vi "Main.vi"() -> ()   [LabVIEW 2010]
uses:
  <vilib>/Platform/storage/lvStorage.llb/xStorage/Open Data Storage/Open Data Storage.xnode
  <vilib>/Platform/storage/lvStorage.llb/xStorage/Set Properties/Set Properties.xnode
  <vilib>/Platform/storage/lvStorage.llb/xStorage/Write Data/Write Data.xnode
  <vilib>/Platform/storage/Storage.llb/usiOverwriteOptions.ctl
  <vilib>/Platform/storage/Storage.llb/usiSequenceRepresentation.ctl
  <vilib>/Platform/storage/lvStorage.llb/xStorage/Close Data Storage/Close Data Storage.xnode
  <instrlib>/Tektronix DPO MSO 2000 4000 Series/Public/Data/Read (Single Waveform).vi
  <instrlib>/Tektronix DPO MSO 2000 4000 Series/Public/Data/Read (Multiple Waveforms).vi
  <instrlib>/Tektronix DPO MSO 2000 4000 Series/Public/Configure/Configure Math (Dual).vi
  <vilib>/Platform/storage/lvStorage.llb/_openStorageWithRootAutoDetect.vi
  <vilib>/Platform/storage/lvStorage.llb/xStorage/xStorageSupp/ErrorOut.vi
  <vilib>/Platform/storage/Storage.llb/__savePropString.vi
  <vilib>/Platform/storage/Storage.llb/__savePropTime.vi
  <vilib>/Platform/storage/lvStorage.llb/_createOrGetByNameExplicitChildObject.vi
  <vilib>/Platform/storage/lvStorage.llb/_prepDDT.vi
  <vilib>/Platform/storage/lvStorage.llb/_getChannelNameFromDDT.vi
  <vilib>/Platform/storage/lvStorage.llb/_saveDDT.vi
  <vilib>/Platform/storage/Storage.llb/Get Object Info.vi
  <vilib>/Platform/storage/Storage.llb/__closeStorageFromObject.vi
  <instrlib>/Tektronix DPO MSO 2000 4000 Series/Tektronix DPO MSO 2000 4000 Series.lvlib
  user32.dll
  shell32.dll
panel:
  out "error out 8":errorcluster
  in  "stop 2":bool
  out "error out 7":errorcluster
  out "error out 6":errorcluster
  in  "stop":bool
  out "Array 5":dbl[](array[numeric])
  out "Array 4":dbl[](array[numeric])
  out "Array 3":dbl[](array[numeric])
  out "Array 2":dbl[](array[numeric])
  out "error out 5":errorcluster
  out "error out 4":errorcluster
  out "ERROR":bool
  in  "Parameters":string
  out "Array":string[](array[string])
  out "error out 2":errorcluster
  out "error out":errorcluster
  out "down":bool
  out "up":bool
  out "DOWN":dbl
  out "UP":dbl
  in  "Error Range":dbl min=0.0 max=5.0 step=0.1 format="%#.3g%"
  in  "Port to test":u16(ring) items=["AMB 1", "AMB 2", "AMB 3", "AMB 4", "AMB 5", "AMB 18"]
  in  "Assembled by":string="Alexis Ibarra"
  in  "ABM-S/N":string
  in  "IP Addres":string
  in  "Tab Control":T1(tab)
  in  "Start TE TEST":bool
  out "TIMA":waveform(dbl)(graph)
  out "TIMB":waveform(dbl)(graph)
  out "Differential Signal":waveform(dbl)(graph)
  out "TE Signals":waveform(dbl)[](graph)
  in  "Maximum Time (10000ms)":u32=20000
  in  "Channel B (1: Channel 2)":u16(ring)=1 items=["Channel 1", "Channel 2", "Channel 3", "Channel 4", "Math", "Reference 1", "Reference 2", "Reference 3", "Reference 4"]
  in  "Channel A (0: Channel 1)":u16(ring) items=["Channel 1", "Channel 2", "Channel 3", "Channel 4", "Math", "Reference 1", "Reference 2", "Reference 3", "Reference 4"]
  out "TE Periode":dbl
  out "TE Average":dbl
  out "TE STATUS":string
  out "TE Amplitude":dbl format="%#_gv"
  in  "Start CCT TEST":bool
  out "TIMB 2":waveform(dbl)(graph)
  out "CAN Diferential":waveform(dbl)(graph)
  out "CAN+TIMB":waveform(dbl)[](graph)
  in  "Maximum Time (10000ms) t2":u32=20000
  in  "Channel B (1: Channel 2) 2":u16(ring)=1 items=["Channel 1", "Channel 2", "Channel 3", "Channel 4", "Math", "Reference 1", "Reference 2", "Reference 3", "Reference 4"]
  in  "Channel A (0: Channel 1) 2":u16(ring) items=["Channel 1", "Channel 2", "Channel 3", "Channel 4", "Math", "Reference 1", "Reference 2", "Reference 3", "Reference 4"]
  out "CCT Delay":dbl format="%^#_6gs"
  out "CCT Average":dbl format="%#_gms"
  out "CCT STATUS":string
  out "Amplitude":dbl format="%#_gv"
  in  "Start CSMT TEST":bool
  out "CAN+TIMB 2":waveform(dbl)(graph)
  out "TIMB 3":waveform(dbl)(graph)
  out "CAN Diferential 2":waveform(dbl)(graph)
  out "CSMT Averege":dbl
  out "CSMT Periode":dbl
  out "CSMT Status":string
  in  "Maximum Time (10000ms) 2":u32=20000
  in  "Channel B (1: Channel 2) 3":u16(ring)=1 items=["Channel 1", "Channel 2", "Channel 3", "Channel 4", "Math", "Reference 1", "Reference 2", "Reference 3", "Reference 4"]
  in  "Channel A (0: Channel 1) 3":u16(ring) items=["Channel 1", "Channel 2", "Channel 3", "Channel 4", "Math", "Reference 1", "Reference 2", "Reference 3", "Reference 4"]
  out "Amplitude":dbl format="%#_gv"
  in  "Start RESET TEST":bool
  out "RESA+RESB":waveform(dbl)[](graph)
  out "RESB":waveform(dbl)(graph)
  out "RESA":waveform(dbl)(graph)
  in  "Channel B (1: Channel 2) 4":u16(ring)=1 items=["Channel 1", "Channel 2", "Channel 3", "Channel 4", "Math", "Reference 1", "Reference 2", "Reference 3", "Reference 4"]
  in  "Channel A (0: Channel 1) 4":u16(ring) items=["Channel 1", "Channel 2", "Channel 3", "Channel 4", "Math", "Reference 1", "Reference 2", "Reference 3", "Reference 4"]
  in  "Maximum Time (10000ms) 3":u32=20000
  out "average":dbl
  out "STATUS":string
  out "Delay":dbl format="%^#_6g"
  out "Amplitude":dbl format="%#_gv"
  in  "AMBSI 1 SERIAL NUMBER":string
  out "Output":string
  in  "Start CM test":bool
  out "Error":string
  in  "?":bool
  in  "?":bool
  in  "Enter ABM Serial Number":string
  in  "Reports":i32(listbox)=-1
  out "output param":i32
  in  "error in":errorcluster
  out "error out 3":errorcluster
  in  "?":bool
  # "ABM Verification System"
  # "Copyrigth Alexis Ibarrra -  ALMA  Computing"
  # "TE Test"
  # "Can Control Timming"
  # "Can Signals Monitoring Timming"
  # "Reset Signal"
  # "Search Reports"
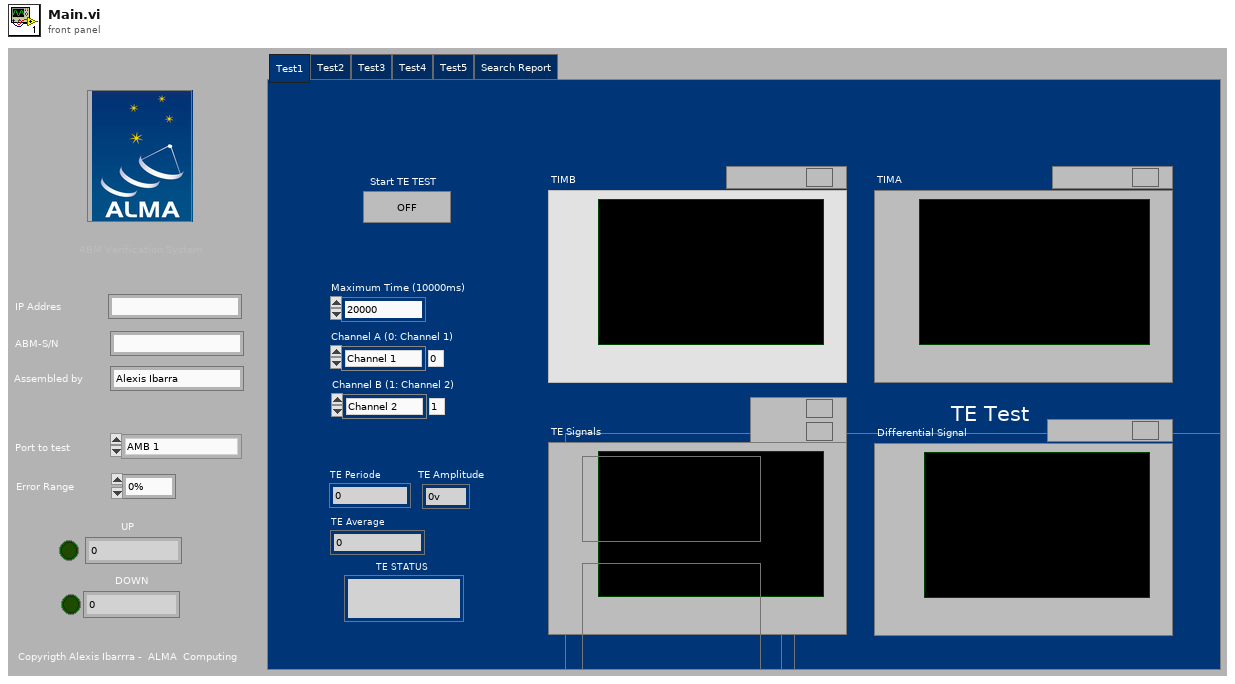
[diagram p1: front panel]
types:
  T1 = enum32{"Test1", "Test2", "Test3", "Test4", "Test5", "Search Report"}
  T2 = enum32{"invalid app kind", "Development System", "Run Time System", "Student Edition", "Embedded LabVIEW", "Evaluation", "Custom"}
  T3 = enum16{"open", "open or create", "create or replace", "create", "open (read only)"}
  T4 = enum16{"UPDATE", "READ", "QUERY", "CREATE CHILD", "CREATE", "CONNECT", "DISCONNECT"}
  T5 = typedef "usiOverwriteOptions.ctl" = enum16{"Append values", "Replace values at index", "Replace all values", "Append if timeline aligns"}
  T6 = typedef "usiSequenceRepresentation.ctl" = enum16{"explicit", "implicit"}
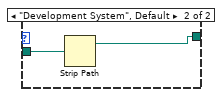
[diagram p3: hidden frame]
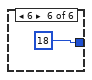
[diagram p8: hidden frame]
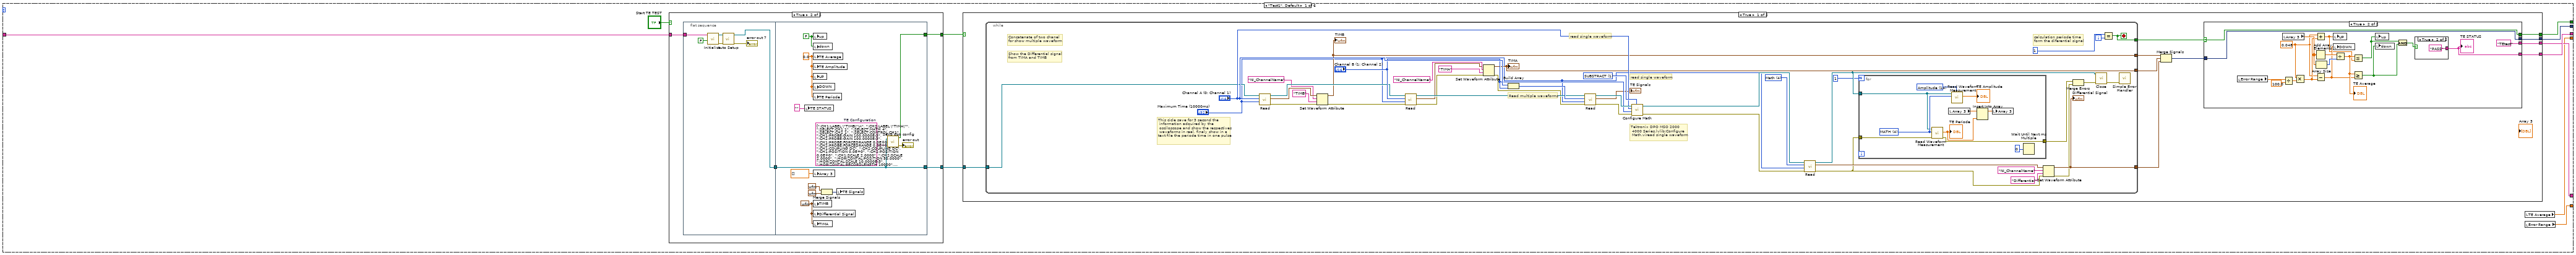
[diagram p9: hidden frame]
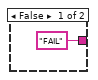
[diagram p11: hidden frame]
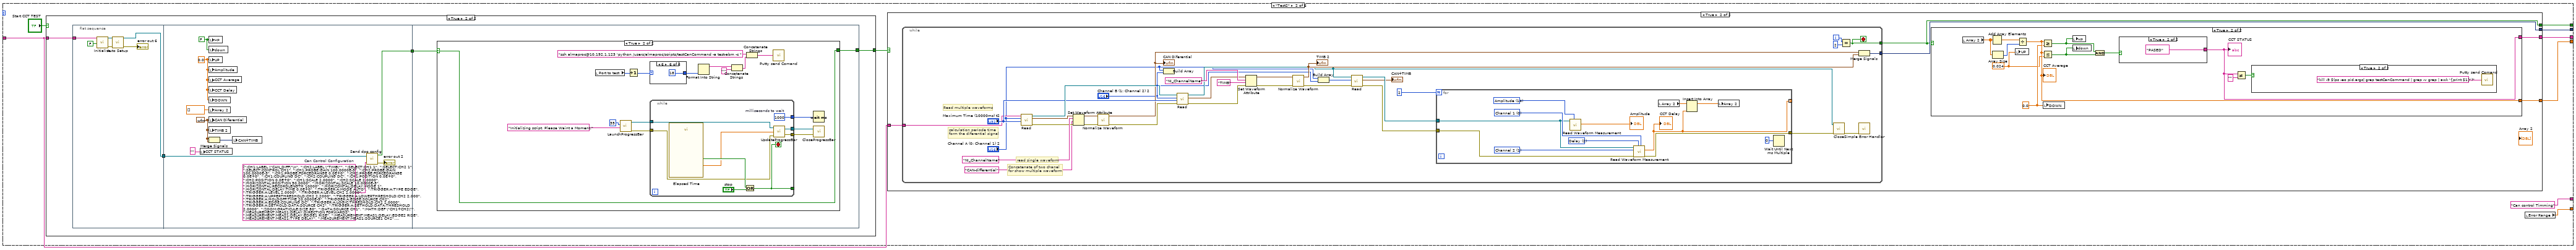
[diagram p14: hidden frame]
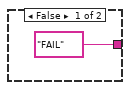
[diagram p18: hidden frame]
diagram:
  # "10.195.18.178"
  n1 = Concatenate Strings("TCPIP0::", "IP Addres", "::inst0::INSTR") -> (w2:string)
  n2 = case shown="\"Test3\"" "Tab Control" {
    tunnel: w2 -> [w19 w125 w251 w387 _ _]
    tunnel: [w18 w131 w254 w378 _ _] -> w1
    tunnel: [w17 w130 w257 w385 _ _] -> w7
    tunnel: [w16 w129 w255 w384 _ _] -> w6
    tunnel: [w12 w126 w252 w382 _ _] -> w5
    tunnel: [w13 w127 w253 w383 _ _] -> w4
    tunnel: [w15 "Can control Timming" "Can SIgnal Monitoring Timming" "Reset  test" _ _] -> w3
    frame "Test1", Default {
      n3 = case shown="True" "Start TE TEST" {
        tunnel: w19 -> [_ w105]
        tunnel: [_ w102] -> w20
        tunnel: [_ w103] -> w14
        frame False {
        }
        frame True {
          n4 = flat-sequence {
            tunnel: w105 -> [w108]
            tunnel: [w107] -> w104
            tunnel: w104 -> [w115]
            tunnel: [w115] -> w103
            tunnel: [w112] -> w102
            frame #0 {
              n5 = call <instrlib>:"Initialize.vi"("Reset (True)"=FALSE, "VISA resource name"=w108) -> ("error out"=w110:errorcluster, "VISA resource name out"=w109:refnum<visa-resource-name>)  [unwired: 8 in]
              n6 = call <instrlib>:"Auto Setup.vi"("error in (no error)"=w110, "VISA resource name"=w109) -> ("error out"=→"error out 7":errorcluster, "VISA resource name out"=w107:refnum<visa-resource-name>)  [unwired: 8 in]
            }
            frame #1 {
              w119 = waveform(dbl) {"t0"=timestamp(0 s since 1904-01-01), "dt"=1.0, "Y"=[]} ("Waveform")
              w123 = 0.0
              w117 = FALSE
              w114 = string[] [":CH1:LABEL \"TIMB\"\n", ":CH2:LABEL \"TIMA\"", ":SELECT:CH1 1", ":SELECT:MATH 4", ":SELECT:CH2 1", ":SELECT:CONTROL CH1", ":CH1:PROBE:GAIN 100.0000E-3", ":CH2:PROBE:GAIN 100.0000E-3", ":CH1:PROBE:FORCEDRANGE 0.0E+0", ":CH2:PROBE:FORCEDRANGE 0.0E+0", ":CH1:COUPLING DC", ":CH2:COUPLING DC", ":CH1:POSITION 0.0E+0", ":CH2:POSITION 0.0E+0", ":CH1:SCALE 2.0000", ":CH2:SCALE 2.0000", ":HORIZONTAL:POSITION 50.0000", ":HORIZONTAL:SCALE 10.0000E-3", ":HORIZONTAL:RECORDLENGTH 10000", ":HORIZONTAL:DELAY:MODE 1", ":HORIZONTAL:DELAY:TIME 0.0E+0", ":TRIGGER:A:MODE AUTO", ":TRIGGER:A:TYPE EDGE", ":TRIGGER:A:LEVEL 2.0000", ":TRIGGER:A:LEVEL:CH2 2.0000", ":TRIGGER:A:UPPERTHRESHOLD:CH2 2.2000", ":TRIGGER:A:LOWERTHRESHOLD:CH2 2.000", ":TRIGGER:A:HOLDOFF:TIME 20.0000E-9", ":TRIGGER:A:EDGE:SOURCE CH2", ":TRIGGER:A:EDGE:COUPLING DC", ":TRIGGER:A:LOGIC:THRESHOLD:CH2 2.0000", ":TRIGGER:A:SETHOLD:DATA:SOURCE CH2", ":TRIGGER:A:SETHOLD:DATA:THRESHOLD 2.0000", ":ZOOM:GRATICULE:SIZE 80", ":DATA:SOURCE CH2", ":MATH:POSITION -3.00E-3", ":MATH:SCALE 2.0000"]  # TE Configuration
              n7 = local write "TE STATUS"("" ("TE STATUS")) -> ()
              n8 = local write "up"(w117) -> ()
              n9 = local write "down"(w117) -> ()
              n10 = local write "TE Average"(w123) -> ()
              n11 = local write "TE Amplitude"(w123) -> ()
              n12 = local write "UP"(w123) -> ()
              n13 = local write "DOWN"(w123) -> ()
              n14 = local write "TE Periode"(w123) -> ()
              n15 = local write "Array 3"(dbl[] []) -> ()
              n16 = local write "TIMB"(w119) -> ()
              n17 = local write "Differential Signal"(w119) -> ()
              n18 = local write "TIMA"(w119) -> ()
              n19 = Merge Signals(waveform(dbl) {"t0"=timestamp(0 s since 1904-01-01), "dt"=1.0, "Y"=[]} ("Waveform"), waveform(dbl) {"t0"=timestamp(0 s since 1904-01-01), "dt"=1.0, "Y"=[]} ("Waveform")) -> (w122:dynamicdata)
              n20 = local write "TE Signals"(w122) -> ()
              n21 = call "Send dpo config.vi"("Array Configuration"=w114, "TCP/IP Addres"=w115) -> ("error out"=→"error out":errorcluster, "Exit"=w112:bool)  [unwired: 1 out]
            }
          }
        }
      }
      n22 = case shown="True" w20 {
        tunnel: w14 -> [w28 _]
        tunnel: [w24 _] -> w18
        tunnel: [w26 _] -> w17
        tunnel: [w23 _] -> w16
        tunnel: [w22 _] -> w15
        frame True {
          n23 = while {
            tunnel: [w65] -> w31
            tunnel: w28 -> [w80]
            tunnel: [w77] -> w29
            tunnel: [w69] -> w30
            tunnel: [w52] -> w25
            i -> [w55]
            stop <- w52 stop-if-true
            w61 = u16 4 items=["Channel 1", "Channel 2", "Channel 3", "Channel 4", "Math", "Reference 1", "Reference 2", "Reference 3", "Reference 4"] ("Channel (0: Channel 1)")
            w88 = u16 1 items=["ADD", "SUBSTRACT", "MULTIPLY", "DIVIDE"] ("Operator (0: ADD)")
            # "This cicle save for 3 second the\n information adquired by the\n osciloscope and show the respectives\n waveforms in real, finaly show in a \ntext file the periode time in one pulse"
            # "Concatenate of two chanel \nfor show multiple waveform"
            # "read single waveform"
            # "read single waveform"
            # "Tektronix DPO MSO 2000\n 4000 Series.lvlib:Configure\n Math.viread single waveform"
            # "calculation periode time\nform the diferential signal"
            # "Show the Differential signal \nfrom TIMA and TIMB"
            # "Read multiple waveforms"
            n24 = call-poly <instrlib>:"Read.vi"("Maximum Time (10000ms)"="Maximum Time (10000ms)", "Channel (0: Channel 1)"="Channel A (0: Channel 1)", "VISA resource name"=w80) -> ("error out"=w76:errorcluster, "Waveform Graph"=w79:waveform(dbl), "VISA resource name out"=w82:refnum<visa-resource-name>)  [unwired: 6 in]
            n25 = Set Waveform Attribute(4:w76, 5:"TIMB" ("name"), 6:"NI_ChannelName" ("name"), 7:w79) -> (0:w75:errorcluster, 3:w77:waveform(dbl))  [unwired: 1 out]
            "TIMB" <- w77
            n26 = call-poly <instrlib>:"Read.vi"("error in (no error)"=w75, "Maximum Time (10000ms)"="Maximum Time (10000ms)", "Channel (0: Channel 1)"="Channel B (1: Channel 2)", "VISA resource name"=w82) -> ("error out"=w71:errorcluster, "Waveform Graph"=w72:waveform(dbl), "VISA resource name out"=w81:refnum<visa-resource-name>)  [unwired: 5 in]
            n27 = Set Waveform Attribute(4:w71, 5:"TIMA" ("name"), 6:"NI_ChannelName" ("name"), 7:w72) -> (0:w70:errorcluster, 3:w69:waveform(dbl))  [unwired: 1 out]
            "TIMA" <- w69
            n28 = Build Array("Channel A (0: Channel 1)", "Channel B (1: Channel 2)") -> (w90:u16[])
            n29 = call-poly <instrlib>:"Read.vi"("error in (no error)"=w70, "Maximum Time (10000ms)"="Maximum Time (10000ms)", "Channels"=w90, "VISA resource name"=w81) -> ("error out"=w89:errorcluster, "Waveform Data"=→"TE Signals":waveform(dbl)[], "VISA resource name out"=w86:refnum<visa-resource-name>)  [unwired: 5 in]
            n30 = call-poly <instrlib>:"Configure Math.vi"("Operator (0: ADD)"=w88, "error in (no error)"=w89, "2nd Source (1: Channel 2)"="Channel B (1: Channel 2)", "1st Source (0: Channel 1)"="Channel A (0: Channel 1)", "VISA resource name"=w86) -> ("error out"=w85:errorcluster, "VISA resource name out"=w87:refnum<visa-resource-name>)  [unwired: 5 in]
            n31 = call-poly <instrlib>:"Read.vi"("error in (no error)"=w85, "Maximum Time (10000ms)"="Maximum Time (10000ms)", "Channel (0: Channel 1)"=w61, "VISA resource name"=w87) -> ("error out"=w59:errorcluster, "Waveform Graph"=w66:waveform(dbl), "VISA resource name out"=w60:refnum<visa-resource-name>)  [unwired: 5 in]
            n32 = for {
              N: 1 -> [_]
              tunnel: w60 -> [w92]
              tunnel: w59 -> [w101]
              tunnel: [w99] -> w58
              w94 = 14 items=["Period", "Frequency", "Delay", "Rise Time", "Fall Time", "Positive Duty Cycle", "Negative Duty Cycle", "Positive Pulse Width", "Negative Pulse Width", "Burst Width", "Phase", "Positive Overshoot", "Negative Overshoot", "Vpp", "Amplitude", "Voltage High", "Voltage Low", "Voltage Max", "Voltage Min", "Voltage Mean", "Voltage Mean (cycle)", "Voltage RMS", "Voltage RMS (cycle)", "Area", "Cycle Area", "Positive Edge Count", "Negative Edge Count", "Positive Pulse Count", "Negative Pulse Count"] ("Measurement Function (0: Period)")
              w93 = u16 4 items=["Channel 1", "Channel 2", "Channel 3", "Channel 4", "MATH", "Reference 1", "Reference 2", "Reference 3", "Reference 4"] ("Channel (0: Channel 1)")
              n33 = call <instrlib>:"Read Waveform Measurement.vi"("error in (no error)"=w101, "Channel (0: Channel 1)"=w93, "VISA resource name"=w92) -> ("error out"=w99:errorcluster, "Measurement Value"=w98:dbl)  [unwired: 6 in, 1 out]
              "TE Periode" <- w98
              n34 = local read "Array 3"() -> (w97:dbl[])
              n35 = call <instrlib>:"Read Waveform Measurement.vi"("Measurement Function (0: Period)"=w94, "Channel (0: Channel 1)"=w93, "VISA resource name"=w92) -> ("Measurement Value"=→"TE Amplitude":dbl)  [unwired: 6 in, 2 out]
              n36 = Insert Into Array(array=w97, new element=w98) -> (w96:dbl[])  [unwired: 1 in]
              n37 = local write "Array 3"(w96) -> ()
              n38 = Wait Until Next ms Multiple(millisecond multiple=u32 0) -> ()  [unwired: 1 out]
            }
            n39 = Set Waveform Attribute(4:w59, 5:"Differential" ("name"), 6:"NI_ChannelName" ("name"), 7:w66) -> (0:w57:errorcluster, 3:w65:waveform(dbl))  [unwired: 1 out]
            "Differential Signal" <- w65
            n40 = Merge Errors(w58, w57) -> (w56:errorcluster)
            n41 = call <instrlib>:"Close.vi"("error in (no error)"=w56, "VISA resource name"=w60) -> ("error out"=w91:errorcluster)  [unwired: 9 in]
            n42 = Equal?(x=1, y=w55) -> (x = y?=w52:bool)
            n43 = call <vilib>:"Simple Error Handler.vi"("error in (no error)"=w91) -> ()  [unwired: 4 in, 5 out]
          }
          n44 = Merge Signals "Merge Signals"(w29, w30, w31) -> (w27:dynamicdata)
          n45 = case shown="True" w25 {
            selector: w25 -> [_ w34]
            tunnel: w27 -> [_ w35]
            tunnel: [_ w35] -> w26
            tunnel: [_ w34] -> w24
            tunnel: [_ w33] -> w23
            tunnel: [_ "TEtest"] -> w22
            frame False {
            }
            frame True {
              w38 = 0.048 ("x")
              n46 = local read "Error Range"() -> (w41:dbl)
              n47 = local read "Array 3"() -> (w47:dbl[])
              n48 = Divide(x=w41, y=100.0) -> (x/y=w37:dbl)
              n49 = Multiply(x=w38, y=w37) -> (x*y=w39:dbl)
              n50 = Add Array Elements(numeric array=w47) -> (sum=w46:dbl)
              n51 = Add(x=w38, y=w39) -> (x+y=w42:dbl)
              n52 = Subtract(x=w38, y=w39) -> (x-y=w43:dbl)
              n53 = Array Size(array=w47) -> (size(s)=w48:i32)
              n54 = local write "UP"(w42) -> ()
              n55 = local write "DOWN"(w43) -> ()
              n56 = Divide(x=w46, y=w48) -> (x/y=w49:dbl)
              "TE Average" <- w49
              n57 = Less Or Equal?(x=w49, y=w42) -> (x <= y?=w44:bool)
              n58 = Greater Or Equal?(x=w49, y=w43) -> (x >= y?=w45:bool)
              n59 = local write "up"(w44) -> ()
              n60 = local write "down"(w45) -> ()
              n61 = And(x=w44, y=w45) -> (x .and. y?=w40:bool)
              n62 = case shown="True" w40 {
                tunnel: ["FAIL" "PASS"] -> w33
                frame False {
                }
                frame True {
                }
              }
              "TE STATUS" <- w33
            }
          }
        }
        frame False {
        }
      }
      n63 = local read "TE Average"() -> (w12:dbl)
      n64 = local read "Error Range"() -> (w13:dbl)
    }
    frame "Test2" {
      n65 = case shown="True" "Start CCT TEST" {
        tunnel: w125 -> [_ w201]
        tunnel: [_ w199] -> w124
        frame False {
        }
        frame True {
          n66 = flat-sequence {
            tunnel: w201 -> [w204]
            tunnel: [w203] -> w200
            tunnel: w200 -> [w211]
            tunnel: [w208] -> w198
            tunnel: [w218] -> w199
            tunnel: w198 -> [w219]
            frame #0 {
              n67 = call <instrlib>:"Initialize.vi"("Reset (True)"=FALSE, "VISA resource name"=w204) -> ("error out"=w206:errorcluster, "VISA resource name out"=w205:refnum<visa-resource-name>)  [unwired: 8 in]
              n68 = call <instrlib>:"Auto Setup.vi"("error in (no error)"=w206, "VISA resource name"=w205) -> ("error out"=→"error out 6":errorcluster, "VISA resource name out"=w203:refnum<visa-resource-name>)  [unwired: 8 in]
            }
            frame #1 {
              w212 = 0.0
              w217 = waveform(dbl) {"t0"=timestamp(0 s since 1904-01-01), "dt"=1.0, "Y"=[]} ("Waveform")
              w214 = FALSE
              w210 = string[] [":CH1:LABEL \"CAN_DIFF\"\n", ":CH2:LABEL \"TIMB\"", ":SELECT:CH1 1", ":SELECT:CH2 1", ":SELECT:CONTROL CH1", ":CH1:PROBE:GAIN 100.0000E-3", ":CH2:PROBE:GAIN 100.0000E-3", ":CH1:PROBE:FORCEDRANGE 0.0E+0", ":CH2:PROBE:FORCEDRANGE 0.0E+0", ":CH1:COUPLING DC", ":CH2:COUPLING DC", ":CH1:POSITION 0.0E+0", ":CH2:POSITION 0.0E+0", ":CH1:SCALE 2.0000", ":CH2:SCALE 2.0000", ":HORIZONTAL:POSITION 50.0000", ":HORIZONTAL:SCALE 10.0000E-3", ":HORIZONTAL:RECORDLENGTH 10000", ":HORIZONTAL:DELAY:MODE 1", ":HORIZONTAL:DELAY:TIME 0.0E+0", ":TRIGGER:A:MODE AUTO", ":TRIGGER:A:TYPE EDGE", ":TRIGGER:A:LEVEL 2.0000", ":TRIGGER:A:LEVEL:CH2 2.0000", ":TRIGGER:A:UPPERTHRESHOLD:CH2 2.2000", ":TRIGGER:A:LOWERTHRESHOLD:CH2 2.000", ":TRIGGER:A:HOLDOFF:TIME 20.0000E-9", ":TRIGGER:A:EDGE:SOURCE CH2", ":TRIGGER:A:EDGE:COUPLING DC", ":TRIGGER:A:LOGIC:THRESHOLD:CH2 2.0000", ":TRIGGER:A:SETHOLD:DATA:SOURCE CH2", ":TRIGGER:A:SETHOLD:DATA:THRESHOLD 2.0000", ":ZOOM:GRATICULE:SIZE 80", ":DATA:SOURCE CH1", ":MATH:DEF \"CH1+CH2\"", ":MEASUREMENT:MEAS1:DELAY:DIRECTION FORWARDS", ":MEASUREMENT:MEAS1:DELAY:EDGE1 RISE", ":MEASUREMENT:MEAS1:DELAY:EDGE2 RISE", ":MEASUREMENT:MEAS1:TYPE DELAY", ":MEASUREMENT:MEAS1:SOURCE1 CH2", ":MEASUREMENT:MEAS1:SOURCE2 CH1", ":MEASUREMENT:MEAS1:STATE 1"]  # Can Control Configuration
              n69 = local write "CCT STATUS"("" ("TE STATUS")) -> ()
              n70 = local write "up"(w214) -> ()
              n71 = local write "down"(w214) -> ()
              n72 = local write "UP"(w212) -> ()
              n73 = local write "Amplitude"(w212) -> ()
              n74 = local write "CCT Average"(w212) -> ()
              n75 = local write "CCT Delay"(w212) -> ()
              n76 = local write "DOWN"(w212) -> ()
              n77 = local write "Array 2"(dbl[] []) -> ()
              n78 = local write "CAN Diferential"(w217) -> ()
              n79 = local write "TIMB 2"(w217) -> ()
              n80 = Merge Signals(w217, w217) -> (w215:dynamicdata)
              n81 = local write "CAN+TIMB"(w215) -> ()
              n82 = call "Send dpo config.vi"("Array Configuration"=w210, "TCP/IP Addres"=w211) -> ("error out"=→"error out 2":errorcluster, "Exit"=w208:bool)  [unwired: 1 out]
            }
            frame #2 {
              n83 = case shown="True" w219 {
                selector: w219 -> [_ w220]
                tunnel: [_ w220] -> w218
                frame False {
                }
                frame True {
                  n84 = local read "Port to test"() -> (w221:u16)
                  n85 = call "LaunchProgressBar.vi"("Title"="Initializing script, Please Waint a Moment.", "MaxRange"=35) -> ("error out"=w232:errorcluster, "reference out"=w233:refnum<vi>)  [unwired: 4 in]
                  n86 = Increment(x=w221) -> (x+1=w222:u16)
                  n87 = case shown="6" w222 {
                    selector: w222 -> [w245 w246 w247 w248 w249 _]
                    tunnel: [w245 w246 w247 w248 w249 18] -> w223
                    frame 1, Default {
                    }
                    frame 2 {
                    }
                    frame 3 {
                    }
                    frame 4 {
                    }
                    frame 5 {
                    }
                    frame 6 {
                    }
                  }
                  n88 = while {
                    tunnel: [w242] -> w235
                    tunnel: [w241] -> _
                    tunnel: w233 -> [w240]
                    tunnel: w232 -> [w239]
                    tunnel: [w237] -> w231
                    tunnel: [w236] -> w230
                    stop <- w241 stop-if-true
                    w242 = u32 1000  # milliseconds to wait
                    n89 = call "Elapsed Time"() -> ("Elapsed Time (s)"=w238:dbl, "Time has Elapsed"=w243:bool)  [unwired: 12 in, 6 out]
                    n90 = Or(x=w243, y="stop") -> (x .or. y?=w241:bool)
                    n91 = call "UpdateProgressBar.vi"("error in"=w239, "PBarValue"=w238, "reference in"=w240) -> ("error out"=w236:errorcluster, "reference out"=w237:refnum<vi>)
                  }
                  n92 = Format Into String(w223) -> (resulting string=w225:string)  [unwired: 3 in, 1 out]
                  n93 = Concatenate Strings(w225, "'" ("string")) -> (w227:string)
                  n94 = Concatenate Strings("ssh almaproc@10.192.1.123 'python /users/almaproc/scripts/testCanCommand -a test-abm -c " ("Command(s) to Execute"), w227) -> (w228:string)
                  n95 = call "Putty send Comand.vi"("Command(s) to Execute"=w228) -> ()
                  n96 = Wait (ms)(milliseconds to wait=w235) -> ()  [unwired: 1 out]
                  n97 = call "CloseProgressBar.vi"("error in"=w230, "reference in"=w231) -> ()  [unwired: 1 out]
                }
              }
            }
          }
        }
      }
      n98 = case shown="True" w124 {
        tunnel: w125 -> [_ w137]
        tunnel: [_ w134] -> w130
        tunnel: [_ w135] -> w126
        tunnel: [_ w136] -> w129
        tunnel: [_ w133] -> w131
        frame False {
        }
        frame True {
          n99 = while {
            tunnel: w137 -> [w151]
            tunnel: [w152] -> w134
            tunnel: [w140] -> w133
            i -> [w149]
            stop <- w140 stop-if-true
            # "read single waveform"
            # "Concatenate of two chanel \nfor show multiple waveform"
            # "calculation periode time\nform the diferential signal"
            # "Read multiple waveforms"
            n100 = call-poly <instrlib>:"Read.vi"("Maximum Time (10000ms)"="Maximum Time (10000ms) t2", "Channel (0: Channel 1)"="Channel A (0: Channel 1) 2", "VISA resource name"=w151) -> ("error out"=w167:errorcluster, "Waveform Graph"=w156:waveform(dbl), "VISA resource name out"=w169:refnum<visa-resource-name>)  [unwired: 6 in]
            n101 = Set Waveform Attribute(4:w167, 5:"CAN-differential" ("name"), 6:"NI_ChannelName" ("name"), 7:w156) -> (0:w159:errorcluster, 3:w161:waveform(dbl))  [unwired: 1 out]
            n102 = call <vilib>:"Normalize Waveform.vi"("error in (no error)"=w159, "waveform in"=w161) -> ("error out"=w158:errorcluster, "normalized waveform"=w154:waveform(dbl))  [unwired: 6 in, 2 out]
            "CAN Diferential" <- w154
            n103 = Build Array("Channel A (0: Channel 1) 2", "Channel B (1: Channel 2) 2") -> ()  [unwired: 1 out]
            n104 = call-poly <instrlib>:"Read.vi"("error in (no error)"=w158, "Maximum Time (10000ms)"="Maximum Time (10000ms) t2", "Channel (0: Channel 1)"="Channel B (1: Channel 2) 2", "VISA resource name"=w169) -> ("error out"=w164:errorcluster, "Waveform Graph"=w155:waveform(dbl), "VISA resource name out"=w146:refnum<visa-resource-name>)  [unwired: 5 in]
            n105 = Set Waveform Attribute(4:w164, 5:"TIMB" ("name"), 6:"NI_ChannelName" ("name"), 7:w155) -> (0:w157:errorcluster, 3:w160:waveform(dbl))  [unwired: 1 out]
            n106 = call <vilib>:"Normalize Waveform.vi"("error in (no error)"=w157, "waveform in"=w160) -> ("error out"=w148:errorcluster, "normalized waveform"=w153:waveform(dbl))  [unwired: 6 in, 2 out]
            "TIMB 2" <- w153
            n107 = Build Array("Channel A (0: Channel 1) 2", "Channel B (1: Channel 2) 2") -> (w142:u16[])
            n108 = call-poly <instrlib>:"Read.vi"("error in (no error)"=w148, "Channels"=w142, "VISA resource name"=w146) -> ("error out"=w147:errorcluster, "Waveform Data"=→"CAN+TIMB":waveform(dbl)[], "VISA resource name out"=w145:refnum<visa-resource-name>)  [unwired: 6 in]
            n109 = for {
              N: 2 -> [_]
              tunnel: w145 -> [w173]
              tunnel: [w181] -> w150
              tunnel: w147 -> [w180]
              tunnel: [w175] -> _ mode=indexing
              w172 = 14 items=["Period", "Frequency", "Delay", "Rise Time", "Fall Time", "Positive Duty Cycle", "Negative Duty Cycle", "Positive Pulse Width", "Negative Pulse Width", "Burst Width", "Phase", "Positive Overshoot", "Negative Overshoot", "Vpp", "Amplitude", "Voltage High", "Voltage Low", "Voltage Max", "Voltage Min", "Voltage Mean", "Voltage Mean (cycle)", "Voltage RMS", "Voltage RMS (cycle)", "Area", "Cycle Area", "Positive Edge Count", "Negative Edge Count", "Positive Pulse Count", "Negative Pulse Count"] ("Measurement Function (0: Period)")
              w178 = u16 0 items=["Channel 1", "Channel 2", "Channel 3", "Channel 4", "MATH", "Reference 1", "Reference 2", "Reference 3", "Reference 4"] ("Destination Channel (1: Channel 2)")
              w179 = u16 1 items=["Channel 1", "Channel 2", "Channel 3", "Channel 4", "MATH", "Reference 1", "Reference 2", "Reference 3", "Reference 4"] ("Channel (0: Channel 1)")
              w174 = 2 items=["Period", "Frequency", "Delay", "Rise Time", "Fall Time", "Positive Duty Cycle", "Negative Duty Cycle", "Positive Pulse Width", "Negative Pulse Width", "Burst Width", "Phase", "Positive Overshoot", "Negative Overshoot", "Vpp", "Amplitude", "Voltage High", "Voltage Low", "Voltage Max", "Voltage Min", "Voltage Mean", "Voltage Mean (cycle)", "Voltage RMS", "Voltage RMS (cycle)", "Area", "Cycle Area", "Positive Edge Count", "Negative Edge Count", "Positive Pulse Count", "Negative Pulse Count"] ("Measurement Function (0: Period)")
              n110 = call <instrlib>:"Read Waveform Measurement.vi"("Measurement Function (0: Period)"=w172, "VISA resource name"=w173) -> ("Measurement Value"=→"Amplitude":dbl)  [unwired: 7 in, 2 out]
              n111 = call <instrlib>:"Read Waveform Measurement.vi"("Destination Channel (1: Channel 2)"=w178, "Measurement Function (0: Period)"=w174, "error in (no error)"=w180, "Channel (0: Channel 1)"=w179, "VISA resource name"=w173) -> ("error out"=w181:errorcluster, "Measurement Value"=w175:dbl)  [unwired: 4 in, 1 out]
              "CCT Delay" <- w175
              n112 = local read "Array 2"() -> (w177:dbl[])
              n113 = Insert Into Array(array=w177, new element=w175) -> (w176:dbl[])  [unwired: 1 in]
              n114 = local write "Array 2"(w176) -> ()
              n115 = Wait Until Next ms Multiple(millisecond multiple=u32 0) -> ()  [unwired: 1 out]
            }
            n116 = call <instrlib>:"Close.vi"("error in (no error)"=w150, "VISA resource name"=w146) -> ("error out"=w170:errorcluster)  [unwired: 9 in]
            n117 = Equal?(x=w149, y=2) -> (x = y?=w140:bool)
            n118 = Merge Signals(w154, w153) -> (w152:dynamicdata)
            n119 = call <vilib>:"Simple Error Handler.vi"("error in (no error)"=w170) -> ()  [unwired: 4 in, 5 out]
          }
          n120 = case shown="True" w133 {
            tunnel: [_ w187] -> w136
            tunnel: [_ w193] -> w135
            frame False {
            }
            frame True {
              w183 = 0.024 ("y")
              w184 = 0.0 ("y")
              n121 = local read "Array 2"() -> (w189:dbl[])
              n122 = Add Array Elements(numeric array=w189) -> (sum=w190:dbl)
              n123 = Array Size(array=w189) -> (size(s)=w188:i32)
              n124 = local write "UP"(w183) -> ()
              n125 = Divide(x=w190, y=w188) -> (x/y=w193:dbl)
              "CCT Average" <- w193
              n126 = Greater Or Equal?(x=w193, y=w184) -> (x >= y?=w192:bool)
              n127 = Less Or Equal?(x=w193, y=w183) -> (x <= y?=w191:bool)
              n128 = local write "DOWN"(w184) -> ()
              n129 = local write "up"(w192) -> ()
              n130 = local write "down"(w191) -> ()
              n131 = And(x=w192, y=w191) -> (x .and. y?=w194:bool)
              n132 = case shown="True" w194 {
                tunnel: ["FAIL" "PASED"] -> w187
                frame False {
                }
                frame True {
                }
              }
              "CCT STATUS" <- w187
              n133 = Not Equal?(x=w187, y="") -> (x != y?=w185:bool)
              n134 = case shown="True" w185 {
                frame False {
                }
                frame True {
                  n135 = call "Putty send Comand.vi"("Command(s) to Execute"="kill -9 $(ps -eo pid,args| grep testCanCommand | grep -v grep | awk '{print $1}')") -> ()
                }
              }
            }
          }
        }
      }
      n136 = local read "Error Range"() -> (w127:dbl)
    }
    frame "Test3" {
      n137 = case shown="True" "Start CSMT TEST" {
        tunnel: [_ w328] -> w258
        tunnel: w251 -> [_ w326]
        frame False {
        }
        frame True {
          n138 = flat-sequence {
            tunnel: w326 -> [w330]
            tunnel: [w329] -> w325
            tunnel: [w336] -> w327
            tunnel: w325 -> [w335]
            tunnel: [w346] -> w328
            tunnel: w327 -> [w345]
            frame #0 {
              n139 = call <instrlib>:"Initialize.vi"("Reset (True)"=FALSE, "VISA resource name"=w330) -> ("error out"=w333:errorcluster, "VISA resource name out"=w332:refnum<visa-resource-name>)  [unwired: 8 in]
              n140 = call <instrlib>:"Auto Setup.vi"("error in (no error)"=w333, "VISA resource name"=w332) -> ("error out"=→"error out 8":errorcluster, "VISA resource name out"=w329:refnum<visa-resource-name>)  [unwired: 8 in]
            }
            frame #1 {
              w337 = string[] [":CH1:LABEL \"CAN_DIFF\"\n", ":CH2:LABEL \"TIMB\"", ":SELECT:CH1 1", ":SELECT:CH2 1", ":SEL:MATH 1", ":SELECT:CONTROL CH1", ":CH1:PROBE:GAIN 100.0000E-3", ":CH2:PROBE:GAIN 100.0000E-3", ":CH1:PROBE:FORCEDRANGE 0.0E+0", ":CH2:PROBE:FORCEDRANGE 0.0E+0", ":CH1:COUPLING DC", ":CH2:COUPLING DC", ":CH1:POSITION 0.0E+0", ":CH2:POSITION 0.0E+0", ":CH1:SCALE 2.0000", ":CH2:SCALE 2.0000", ":MATH:VERT:SCA 2.0000", ":MATH:VERT:POS -3.4", ":MATH:HOR:SCA 10.0000E-3", ":MATH:HOR:POS 50.0000", ":HORIZONTAL:POSITION 50.0000", ":HORIZONTAL:SCALE 10.0000E-3", ":HORIZONTAL:RECORDLENGTH 10000", ":HORIZONTAL:DELAY:MODE 1", ":HORIZONTAL:DELAY:TIME 0.0E+0", ":TRIGGER:A:MODE AUTO", ":TRIGGER:A:TYPE EDGE", ":TRIGGER:A:LEVEL 2.0000", ":TRIGGER:A:LEVEL:CH1 2.0000", ":TRIGGER:A:UPPERTHRESHOLD:CH1 2.2000", ":TRIGGER:A:LOWERTHRESHOLD:CH1 2.000", ":TRIGGER:A:HOLDOFF:TIME 20.0000E-9", ":TRIGGER:A:EDGE:SOURCE CH1", ":TRIGGER:A:EDGE:COUPLING DC", ":TRIGGER:A:LOGIC:THRESHOLD:CH2 2.0000", ":TRIGGER:A:SETHOLD:DATA:SOURCE CH1", ":TRIGGER:A:SETHOLD:DATA:THRESHOLD 2.0000", ":ZOOM:GRATICULE:SIZE 80", ":DATA:SOURCE CH1", ":MATH:DEF \"CH1+CH2\""]  # CSMT Configuration
              w341 = waveform(dbl) {"t0"=timestamp(0 s since 1904-01-01), "dt"=1.0, "Y"=[]} ("Waveform")
              w342 = 0.0
              w343 = FALSE
              n141 = local write "CSMT Status"("" ("TE STATUS")) -> ()
              n142 = local write "up"(w343) -> ()
              n143 = local write "down"(w343) -> ()
              n144 = local write "CSMT Periode"(w342) -> ()
              n145 = local write "UP"(w342) -> ()
              n146 = local write "DOWN"(w342) -> ()
              n147 = local write "Amplitude"(w342) -> ()
              n148 = local write "CSMT Averege"(w342) -> ()
              n149 = local write "Array 4"(dbl[] [] ("Array 4")) -> ()
              n150 = local write "TIMB 3"(w341) -> ()
              n151 = local write "CAN Diferential 2"(w341) -> ()
              n152 = Merge Signals(w341, w341) -> (w340:dynamicdata)
              n153 = local write "CAN+TIMB 2"(w340) -> ()
              n154 = call "Send dpo config.vi"("Array Configuration"=w337, "TCP/IP Addres"=w335) -> ("error out"=→"error out 4":errorcluster, "Exit"=w336:bool)  [unwired: 1 out]
            }
            frame #2 {
              n155 = case shown="True" w345 {
                selector: w345 -> [_ w347]
                tunnel: [_ w347] -> w346
                frame False {
                }
                frame True {
                  n156 = local read "Port to test"() -> (w348:u16)
                  n157 = call "LaunchProgressBar.vi"("Title"="Initializing script, Please Waint a Moment.", "MaxRange"=35) -> ("error out"=w359:errorcluster, "reference out"=w360:refnum<vi>)  [unwired: 4 in]
                  n158 = Increment(x=w348) -> (x+1=w349:u16)
                  n159 = case shown="6" w349 {
                    selector: w349 -> [w372 w373 w374 w375 w376 _]
                    tunnel: [w372 w373 w374 w375 w376 18] -> w350
                    frame 1, Default {
                    }
                    frame 2 {
                    }
                    frame 3 {
                    }
                    frame 4 {
                    }
                    frame 5 {
                    }
                    frame 6 {
                    }
                  }
                  n160 = while {
                    tunnel: [w369] -> w362
                    tunnel: [w368] -> _
                    tunnel: w360 -> [w367]
                    tunnel: w359 -> [w366]
                    tunnel: [w364] -> w358
                    tunnel: [w363] -> w357
                    stop <- w368 stop-if-true
                    w369 = u32 1000  # milliseconds to wait
                    n161 = call "Elapsed Time2"() -> ("Elapsed Time (s)"=w365:dbl, "Time has Elapsed"=w370:bool)  [unwired: 12 in, 6 out]
                    n162 = Or(x=w370, y="stop 2") -> (x .or. y?=w368:bool)
                    n163 = call "UpdateProgressBar.vi"("error in"=w366, "PBarValue"=w365, "reference in"=w367) -> ("error out"=w363:errorcluster, "reference out"=w364:refnum<vi>)
                  }
                  n164 = Format Into String(w350) -> (resulting string=w352:string)  [unwired: 3 in, 1 out]
                  n165 = Concatenate Strings(w352, "'" ("string")) -> (w354:string)
                  n166 = Concatenate Strings("ssh almaproc@10.192.1.123 'python /users/almaproc/scripts/testCanMonitor -a test-abm -c " ("Command(s) to Execute"), w354) -> (w355:string)
                  n167 = call "Putty send Comand.vi"("Command(s) to Execute"=w355) -> ()
                  n168 = Wait (ms)(milliseconds to wait=w362) -> ()  [unwired: 1 out]
                  n169 = call "CloseProgressBar.vi"("error in"=w357, "reference in"=w358) -> ()  [unwired: 1 out]
                }
              }
            }
          }
        }
      }
      n170 = case shown="True" w258 {
        tunnel: [_ w264] -> w257
        tunnel: [_ w261] -> w254
        tunnel: [_ w263] -> w252
        tunnel: [_ w262] -> w255
        tunnel: w251 -> [_ w260]
        frame False {
        }
        frame True {
          n171 = while {
            tunnel: [w292] -> w264
            tunnel: [w283] -> w261
            tunnel: w260 -> [w280]
            i -> [w284]
            stop <- w283 stop-if-true
            w288 = u16 4 items=["Channel 1", "Channel 2", "Channel 3", "Channel 4", "Math", "Reference 1", "Reference 2", "Reference 3", "Reference 4"] ("Channel (0: Channel 1)")
            # "read single waveform"
            # "Concatenate of two chanel \nfor show multiple waveform"
            # "calculation periode time\nform the diferential signal"
            # "Read multiple waveforms"
            n172 = call-poly <instrlib>:"Read.vi"("Maximum Time (10000ms)"="Maximum Time (10000ms) 2", "Channel (0: Channel 1)"="Channel A (0: Channel 1) 3", "VISA resource name"=w280) -> ("error out"=w309:errorcluster, "Waveform Graph"=w296:waveform(dbl), "VISA resource name out"=w311:refnum<visa-resource-name>)  [unwired: 6 in]
            n173 = Set Waveform Attribute(4:w309, 5:"CAN-differential" ("name"), 6:"NI_ChannelName" ("name"), 7:w296) -> (0:w299:errorcluster, 3:w301:waveform(dbl))  [unwired: 1 out]
            n174 = call <vilib>:"Normalize Waveform.vi"("error in (no error)"=w299, "waveform in"=w301) -> ("error out"=w298:errorcluster, "normalized waveform"=w294:waveform(dbl))  [unwired: 6 in, 2 out]
            "CAN Diferential 2" <- w294
            n175 = Build Array("Channel A (0: Channel 1) 3", "Channel B (1: Channel 2) 3") -> ()  [unwired: 1 out]
            n176 = call-poly <instrlib>:"Read.vi"("error in (no error)"=w298, "Maximum Time (10000ms)"="Maximum Time (10000ms) 2", "Channel (0: Channel 1)"="Channel B (1: Channel 2) 3", "VISA resource name"=w311) -> ("error out"=w306:errorcluster, "Waveform Graph"=w295:waveform(dbl), "VISA resource name out"=w290:refnum<visa-resource-name>)  [unwired: 5 in]
            n177 = Set Waveform Attribute(4:w306, 5:"TIMB" ("name"), 6:"NI_ChannelName" ("name"), 7:w295) -> (0:w297:errorcluster, 3:w300:waveform(dbl))  [unwired: 1 out]
            n178 = call <vilib>:"Normalize Waveform.vi"("error in (no error)"=w297, "waveform in"=w300) -> ("error out"=w291:errorcluster, "normalized waveform"=w293:waveform(dbl))  [unwired: 6 in, 2 out]
            "TIMB 3" <- w293
            n179 = call-poly <instrlib>:"Read.vi"("error in (no error)"=w291, "Channel (0: Channel 1)"=w288, "VISA resource name"=w290) -> ("error out"=w286:errorcluster, "Waveform Graph"=→"CAN+TIMB 2":waveform(dbl), "VISA resource name out"=w285:refnum<visa-resource-name>)  [unwired: 6 in]
            n180 = for {
              N: 3 -> [_]
              tunnel: w285 -> [w314]
              tunnel: [w323] -> w287
              tunnel: w286 -> [w322]
              w313 = u16 0 items=["Channel 1", "Channel 2", "Channel 3", "Channel 4", "MATH", "Reference 1", "Reference 2", "Reference 3", "Reference 4"] ("Destination Channel (1: Channel 2)")
              w315 = 14 items=["Period", "Frequency", "Delay", "Rise Time", "Fall Time", "Positive Duty Cycle", "Negative Duty Cycle", "Positive Pulse Width", "Negative Pulse Width", "Burst Width", "Phase", "Positive Overshoot", "Negative Overshoot", "Vpp", "Amplitude", "Voltage High", "Voltage Low", "Voltage Max", "Voltage Min", "Voltage Mean", "Voltage Mean (cycle)", "Voltage RMS", "Voltage RMS (cycle)", "Area", "Cycle Area", "Positive Edge Count", "Negative Edge Count", "Positive Pulse Count", "Negative Pulse Count"] ("Measurement Function (0: Period)")
              w321 = 2 items=["Period", "Frequency", "Delay", "Rise Time", "Fall Time", "Positive Duty Cycle", "Negative Duty Cycle", "Positive Pulse Width", "Negative Pulse Width", "Burst Width", "Phase", "Positive Overshoot", "Negative Overshoot", "Vpp", "Amplitude", "Voltage High", "Voltage Low", "Voltage Max", "Voltage Min", "Voltage Mean", "Voltage Mean (cycle)", "Voltage RMS", "Voltage RMS (cycle)", "Area", "Cycle Area", "Positive Edge Count", "Negative Edge Count", "Positive Pulse Count", "Negative Pulse Count"] ("Measurement Function (0: Period)")
              w316 = u16 1 items=["Channel 1", "Channel 2", "Channel 3", "Channel 4", "MATH", "Reference 1", "Reference 2", "Reference 3", "Reference 4"] ("Channel (0: Channel 1)")
              n181 = call <instrlib>:"Read Waveform Measurement.vi"("Measurement Function (0: Period)"=w315, "Channel (0: Channel 1)"=w316, "VISA resource name"=w314) -> ("Measurement Value"=→"Amplitude":dbl)  [unwired: 6 in, 2 out]
              n182 = local read "Array 4"() -> (w320:dbl[])
              n183 = call <instrlib>:"Read Waveform Measurement.vi"("Destination Channel (1: Channel 2)"=w313, "Measurement Function (0: Period)"=w321, "error in (no error)"=w322, "Channel (0: Channel 1)"=w316, "VISA resource name"=w314) -> ("error out"=w323:errorcluster, "Measurement Value"=w318:dbl)  [unwired: 4 in, 1 out]
              "CSMT Periode" <- w318
              n184 = Insert Into Array(array=w320, new element=w318) -> (w319:dbl[])  [unwired: 1 in]
              n185 = local write "Array 4"(w319) -> ()
              n186 = Wait Until Next ms Multiple(millisecond multiple=u32 0) -> ()  [unwired: 1 out]
            }
            n187 = call <instrlib>:"Close.vi"("error in (no error)"=w287, "VISA resource name"=w285) -> ("error out"=w312:errorcluster)  [unwired: 9 in]
            n188 = Equal?(x=w284, y=2) -> (x = y?=w283:bool)
            n189 = Merge Signals(w294, w293) -> (w292:dynamicdata)
            n190 = call <vilib>:"Simple Error Handler.vi"("error in (no error)"=w312) -> ()  [unwired: 4 in, 5 out]
          }
          n191 = case shown="True" w261 {
            tunnel: [_ w273] -> w263
            tunnel: [_ w266] -> w262
            frame False {
            }
            frame True {
              w269 = 0.048 ("x")
              w265 = 0.024 ("x")
              n192 = local read "Array 4"() -> (w270:dbl[])
              n193 = Add Array Elements(numeric array=w270) -> (sum=w272:dbl)
              n194 = Array Size(array=w270) -> (size(s)=w271:i32)
              n195 = local write "UP"(w269) -> ()
              n196 = Divide(x=w272, y=w271) -> (x/y=w273:dbl)
              "CSMT Averege" <- w273
              n197 = Greater Or Equal?(x=w273, y=w265) -> (x >= y?=w275:bool)
              n198 = Less Or Equal?(x=w273, y=w269) -> (x <= y?=w274:bool)
              n199 = local write "DOWN"(w265) -> ()
              n200 = local write "down"(w275) -> ()
              n201 = local write "up"(w274) -> ()
              n202 = And(x=w275, y=w274) -> (x .and. y?=w276:bool)
              n203 = case shown="False" w276 {
                tunnel: ["FAIL" "PASED"] -> w266
                frame False {
                }
                frame True {
                }
              }
              "CSMT Status" <- w266
              n204 = Not Equal?(x=w266, y="") -> (x != y?=w267:bool)
              n205 = case shown="True" w267 {
                frame False {
                }
                frame True {
                  n206 = call "Putty send Comand.vi"("Command(s) to Execute"="kill -9 $(ps -eo pid,args| grep testCanMonitor | grep -v grep | awk '{print $1}')") -> ()
                }
              }
            }
          }
        }
      }
      n207 = local read "Error Range"() -> (w253:dbl)
    }
    frame "Test4" {
      n208 = case shown="True" "Start RESET TEST" {
        selector: "Start RESET TEST" -> [_ w458]
        tunnel: [_ w450] -> w386
        tunnel: [_ w458] -> w379
        tunnel: w387 -> [_ w450]
        frame False {
        }
        frame True {
          w455 = waveform(dbl) {"t0"=timestamp(0 s since 1904-01-01), "dt"=1.0, "Y"=[]} ("Waveform")
          w452 = 0.0
          w457 = FALSE
          w451 = string[] [":MESS:SHOW \"Reset Test\"", ":MESSAGE:BOX 271,82,292,114", ":SEL:CH1 1", ":SEL:CH2 1", ":SEL:CONTRO CH1", ":CH1:PRO:GAIN 100.0000E-3", ":CH2:PRO:GAIN 100.0000E-3", ":CH1:POS 0.0E+0", ":CH2:POS 0.0E+0", ":CH1:SCA 2.0000", ":CH2:SCA 2.0000", ":CH1:LAB \"RESA\"", ":CH2:LAB \"RESB\"", ":HOR:POS 50.0000", ":HOR:SCA 2.0000E-3", ":TRIG:A:LEV 2.0000", ":TRIG:A:LEV:CH1 2.0000", ":TRIG:A:LEV:CH2 2.0400", ":TRIG:A:UPP:CH1 2.0000", ":TRIG:A:UPP:CH2 2.2000", ":TRIG:A:LOW:CH1 2.0000", ":TRIG:A:LOW:CH2 2.0400", ":TRIG:A:HOLD:TIM 20.0000E-9", ":TRIG:A:EDGE:SOU CH1", ":TRIG:A:EDGE:COUP DC", ":TRIG:A:LOGI:THR:CH1 2.0000", ":TRIG:A:LOGI:THR:CH2 2.0400", ":TRIG:A:SETH:CLOC:THR 2.0000", ":TRIG:A:SETH:DAT:SOU CH2", ":TRIG:A:SETH:DAT:THR 2.0400", ":MEASU:IMM:DEL:DIR FORW", ":MEASU:IMM:DEL:EDGE1 RIS", ":MEASU:IMM:DEL:EDGE2 RIS", ":MEASU:IMM:TYP DEL", ":MEASU:IMM:SOU1 CH2", ":MEASU:IMM:SOU2 CH1", ":MEASU:MEAS1:DEL:DIR FORW", ":MEASU:MEAS1:DEL:EDGE1 RIS", ":MEASU:MEAS1:DEL:EDGE2 RIS", ":MEASU:MEAS1:TYP DEL", ":MEASU:MEAS1:SOU1 CH2", ":MEASU:MEAS1:SOU2 CH1", ":MEASU:MEAS1:STATE 1", ":DAT:SOU CH1", ":DAT:STAR 1", ":DAT:STOP 10000000", ""]  # Reset Configuration
          n209 = local write "STATUS"("" ("TE STATUS")) -> ()
          n210 = local write "up"(w457) -> ()
          n211 = local write "down"(w457) -> ()
          n212 = local write "UP"(w452) -> ()
          n213 = local write "Delay"(w452) -> ()
          n214 = local write "Array 5"(dbl[] [] ("Array 5")) -> ()
          n215 = local write "RESA"(w455) -> ()
          n216 = local write "RESB"(w455) -> ()
          n217 = local write "average"(w452) -> ()
          n218 = local write "DOWN"(w452) -> ()
          n219 = local write "Amplitude"(w452) -> ()
          n220 = Merge Signals(w455, w455) -> (w454:dynamicdata)
          n221 = local write "RESA+RESB"(w454) -> ()
          n222 = call "Send dpo config.vi"("Array Configuration"=w451, "TCP/IP Addres"=w450) -> ("error out"=→"error out 5":errorcluster)  [unwired: 2 out]
        }
      }
      n223 = case shown="True" w379 {
        tunnel: w386 -> [_ w393]
        tunnel: [_ w392] -> w385
        tunnel: [_ w390] -> w382
        tunnel: [_ w391] -> w384
        tunnel: [_ w388] -> w378
        frame False {
        }
        frame True {
          n224 = while {
            tunnel: w393 -> [w407]
            tunnel: [w408] -> w392
            tunnel: [w394] -> w389
            i -> [w405]
            stop <- w394 stop-if-true
            # "read single waveform"
            # "Concatenate of two chanel \nfor show multiple waveform"
            # "calculation periode time\nform the diferential signal"
            # "Read multiple waveforms"
            n225 = call-poly <instrlib>:"Read.vi"("Maximum Time (10000ms)"="Maximum Time (10000ms) 3", "Channel (0: Channel 1)"="Channel A (0: Channel 1) 4", "VISA resource name"=w407) -> ("error out"=w423:errorcluster, "Waveform Graph"=w412:waveform(dbl), "VISA resource name out"=w425:refnum<visa-resource-name>)  [unwired: 6 in]
            n226 = Set Waveform Attribute(4:w423, 5:"RESA" ("name"), 6:"NI_ChannelName" ("name"), 7:w412) -> (0:w415:errorcluster, 3:w417:waveform(dbl))  [unwired: 1 out]
            n227 = call <vilib>:"Normalize Waveform.vi"("error in (no error)"=w415, "waveform in"=w417) -> ("error out"=w414:errorcluster, "normalized waveform"=w410:waveform(dbl))  [unwired: 6 in, 2 out]
            "RESA" <- w410
            n228 = Build Array("Channel A (0: Channel 1) 4", "Channel B (1: Channel 2) 4") -> ()  [unwired: 1 out]
            n229 = call-poly <instrlib>:"Read.vi"("error in (no error)"=w414, "Maximum Time (10000ms)"="Maximum Time (10000ms) 3", "Channel (0: Channel 1)"="Channel B (1: Channel 2) 4", "VISA resource name"=w425) -> ("error out"=w420:errorcluster, "Waveform Graph"=w411:waveform(dbl), "VISA resource name out"=w402:refnum<visa-resource-name>)  [unwired: 5 in]
            n230 = Set Waveform Attribute(4:w420, 5:"RESB" ("name"), 6:"NI_ChannelName" ("name"), 7:w411) -> (0:w413:errorcluster, 3:w416:waveform(dbl))  [unwired: 1 out]
            n231 = call <vilib>:"Normalize Waveform.vi"("error in (no error)"=w413, "waveform in"=w416) -> ("error out"=w404:errorcluster, "normalized waveform"=w409:waveform(dbl))  [unwired: 6 in, 2 out]
            "RESB" <- w409
            n232 = Build Array("Channel A (0: Channel 1) 4", "Channel B (1: Channel 2) 4") -> (w398:u16[])
            n233 = call-poly <instrlib>:"Read.vi"("error in (no error)"=w404, "Channels"=w398, "VISA resource name"=w402) -> ("error out"=w403:errorcluster, "Waveform Data"=→"RESA+RESB":waveform(dbl)[], "VISA resource name out"=w401:refnum<visa-resource-name>)  [unwired: 6 in]
            n234 = for {
              N: 1 -> [_]
              tunnel: w401 -> [w430]
              tunnel: [w436] -> _
              tunnel: [w437] -> w406
              tunnel: w403 -> [w436]
              w427 = 14 items=["Period", "Frequency", "Delay", "Rise Time", "Fall Time", "Positive Duty Cycle", "Negative Duty Cycle", "Positive Pulse Width", "Negative Pulse Width", "Burst Width", "Phase", "Positive Overshoot", "Negative Overshoot", "Vpp", "Amplitude", "Voltage High", "Voltage Low", "Voltage Max", "Voltage Min", "Voltage Mean", "Voltage Mean (cycle)", "Voltage RMS", "Voltage RMS (cycle)", "Area", "Cycle Area", "Positive Edge Count", "Negative Edge Count", "Positive Pulse Count", "Negative Pulse Count"] ("Measurement Function (0: Period)")
              w429 = u16 0 items=["Channel 1", "Channel 2", "Channel 3", "Channel 4", "MATH", "Reference 1", "Reference 2", "Reference 3", "Reference 4"] ("Destination Channel (1: Channel 2)")
              w428 = u16 1 items=["Channel 1", "Channel 2", "Channel 3", "Channel 4", "MATH", "Reference 1", "Reference 2", "Reference 3", "Reference 4"] ("Channel (0: Channel 1)")
              w435 = 2 items=["Period", "Frequency", "Delay", "Rise Time", "Fall Time", "Positive Duty Cycle", "Negative Duty Cycle", "Positive Pulse Width", "Negative Pulse Width", "Burst Width", "Phase", "Positive Overshoot", "Negative Overshoot", "Vpp", "Amplitude", "Voltage High", "Voltage Low", "Voltage Max", "Voltage Min", "Voltage Mean", "Voltage Mean (cycle)", "Voltage RMS", "Voltage RMS (cycle)", "Area", "Cycle Area", "Positive Edge Count", "Negative Edge Count", "Positive Pulse Count", "Negative Pulse Count"] ("Measurement Function (0: Period)")
              n235 = call <instrlib>:"Read Waveform Measurement.vi"("Destination Channel (1: Channel 2)"=w428, "Measurement Function (0: Period)"=w427, "Channel (0: Channel 1)"=w429, "VISA resource name"=w430) -> ("Measurement Value"=→"Amplitude":dbl)  [unwired: 5 in, 2 out]
              n236 = call <instrlib>:"Read Waveform Measurement.vi"("Destination Channel (1: Channel 2)"=w429, "Measurement Function (0: Period)"=w435, "error in (no error)"=w436, "Channel (0: Channel 1)"=w428, "VISA resource name"=w430) -> ("error out"=w437:errorcluster, "Measurement Value"=w433:dbl)  [unwired: 4 in, 1 out]
              "Delay" <- w433
              n237 = local read "Array 5"() -> (w434:dbl[])
              n238 = Insert Into Array(array=w434, new element=w433) -> (w432:dbl[])  [unwired: 1 in]
              n239 = local write "Array 5"(w432) -> ()
              n240 = Wait Until Next ms Multiple(millisecond multiple=u32 0) -> ()  [unwired: 1 out]
            }
            n241 = call <instrlib>:"Close.vi"("error in (no error)"=w406, "VISA resource name"=w402) -> ("error out"=w426:errorcluster)  [unwired: 9 in]
            n242 = Equal?(x=w405, y=2) -> (x = y?=w394:bool)
            n243 = Merge Signals(w410, w409) -> (w408:dynamicdata)
            n244 = call <vilib>:"Simple Error Handler.vi"("error in (no error)"=w426) -> ()  [unwired: 4 in, 5 out]
          }
          n245 = case shown="True" w389 {
            selector: w389 -> [_ w442]
            tunnel: [_ w446] -> w390
            tunnel: [_ w445] -> w391
            tunnel: [_ w442] -> w388
            frame False {
            }
            frame True {
              n246 = local read "Array 5"() -> (w440:dbl[])
              n247 = Add Array Elements(numeric array=w440) -> (sum=w439:dbl)
              n248 = Array Size(array=w440) -> (size(s)=w441:i32)
              n249 = Divide(x=w439, y=w441) -> (x/y=w446:dbl)
              "average" <- w446
              n250 = Greater Or Equal?(x=w446, y=0.001) -> (x >= y?=w443:bool)
              n251 = case shown="False" w443 {
                tunnel: ["FAIL" "PASED"] -> w445
                frame False {
                }
                frame True {
                }
              }
              "STATUS" <- w445
            }
          }
        }
      }
      n252 = local read "Error Range"() -> (w383:dbl)
    }
    frame "Test5" {
      n253 = case shown="True" "Start CM test" {
        selector: "Start CM test" -> [_ w467]
        frame False {
        }
        frame True {
          w470 = " "  # standard input
          n254 = case shown="True" w467 {
            frame False {
            }
            frame True {
              w497 = "" ("Output")
              n255 = local write "Error"(w497) -> ()
              n256 = property on="Error" class="Str"("Visible"=FALSE) -> ()  [unwired: 2 in, 2 out]
              n257 = local write "Output"(w497) -> ()
            }
          }
          n258 = call "LaunchProgressBar.vi"("Title"="Test In Progress, Please Wait a Moment", "MaxRange"=13000) -> ("error out"=w463:errorcluster, "reference out"=w462:refnum<vi>)  [unwired: 4 in]
          n259 = Open Application Reference() -> (3:w478:refnum<vi>)  [unwired: 4 in, 1 out]
          n260 = while {
            tunnel: w462 -> [w510]
            tunnel: w463 -> [w509]
            tunnel: [w505] -> w466
            tunnel: [w504] -> w465
            i -> [w507]
            stop <- w499 stop-if-true
            w501 = "" ("y")
            n261 = local read "Error"() -> (w502:string)
            n262 = local read "Output"() -> (w506:string)
            n263 = Not Equal?(x=w502, y=w501) -> (x != y?=w498:bool)
            n264 = Not Equal?(x=w506, y=w501) -> (x != y?=w500:bool)
            n265 = property on="Error" class="Str"("Visible"=w498) -> ()  [unwired: 2 in, 2 out]
            n266 = Or(x=w500, y=w498) -> (x .or. y?=w499:bool)
            n267 = Increment(x=w507) -> (x+1=w508:i32)
            n268 = Wait Until Next ms Multiple(millisecond multiple=u32 2 ("millisecond timer value")) -> ()  [unwired: 1 out]
            n269 = call "UpdateProgressBar.vi"("error in"=w509, "PBarValue"=w508, "reference in"=w510) -> ("error out"=w504:errorcluster, "reference out"=w505:refnum<vi>)
          }
          n270 = local read "Port to test"() -> (w488:u16)
          n271 = property class="App"(reference=w478) -> ("App.Kind"=w479:T2)  [unwired: 1 in, 2 out]
          n272 = Current VI's Path() -> (path=w480:path)
          n273 = Increment(x=w488) -> (x+1=w489:u16)
          n274 = case shown="\"Run Time System\"" w479 {
            tunnel: w480 -> [w517 w522]
            tunnel: [w518 w521] -> w481
            frame "Run Time System" {
              n275 = Strip Path(path=w517) -> (stripped path=w519:path)  [unwired: 1 out]
              n276 = Strip Path(path=w519) -> (stripped path=w520:path)  [unwired: 1 out]
              n277 = Strip Path(path=w520) -> (stripped path=w518:path)  [unwired: 1 out]
            }
            frame "Development System", Default {
              n278 = Strip Path(path=w522) -> (stripped path=w521:path)  [unwired: 1 out]
            }
          }
          n279 = case shown="6" w489 {
            selector: w489 -> [w511 w512 w513 w514 w515 _]
            tunnel: [w511 w512 w513 w514 w515 18] -> w490
            frame 1, Default {
            }
            frame 2 {
            }
            frame 3 {
            }
            frame 4 {
            }
            frame 5 {
            }
            frame 6 {
            }
          }
          n280 = Format Into String(w490) -> (resulting string=w491:string)  [unwired: 3 in, 1 out]
          n281 = Path To String(path=w481) -> (string=w484:string)
          n282 = call "CloseProgressBar.vi"("error in"=w465, "reference in"=w466) -> ()  [unwired: 1 out]
          n283 = Concatenate Strings(w484, "\\putty\\plink.exe " ("command line")) -> (w483:string)
          n284 = Concatenate Strings("ssh almaproc@10.192.1.123 'python /users/almaproc/scripts/testCanMonitorAndCommand -a test-abm -c " ("Command(s) to Execute"), w491, " -s " ("string"), "AMBSI 1 SERIAL NUMBER", "'" ("string")) -> (w495:string)
          n285 = Concatenate Strings(w483, "root" ("Username"), "@" ("string"), "10.192.1.254" ("Host"), " -ssh", " -pw " ("string"), "new2me" ("Password"), " " ("string"), w495) -> (w477:string)
          n286 = call <vilib>:"System Exec.vi"("run minimized? (F)"=TRUE ("Hide DOS\nWindow?"), "wait until completion? (T)"=TRUE, "standard input"=w470, "command line"=w477) -> ("standard error"=→"Error":string, "standard output"=→"Output":string)  [unwired: 2 in, 4 out]
        }
      }
    }
    frame "Search Report" {
      n287 = case shown="True" "?" {
        frame False {
        }
        frame True {
          n288 = local write "Enter ABM Serial Number"("" ("Enter ABM Serial Number")) -> ()
          n289 = property on="Reports" class="LstBox (strict)"("Item Names"=string[] [] ("array")) -> ()  [unwired: 2 in, 2 out]
        }
      }
      n290 = Open Application Reference() -> (3:w526:refnum<vi>)  [unwired: 4 in, 1 out]
      n291 = property class="App"(reference=w526) -> ("App.Kind"=w525:T2)  [unwired: 1 in, 2 out]
      n292 = Current VI's Path() -> (path=w524:path)
      n293 = case shown="\"Run Time System\"" w525 {
        tunnel: w524 -> [w542 w547]
        tunnel: [w543 w546] -> w523
        frame "Run Time System" {
          n294 = Strip Path(path=w542) -> (stripped path=w544:path)  [unwired: 1 out]
          n295 = Strip Path(path=w544) -> (stripped path=w545:path)  [unwired: 1 out]
          n296 = Strip Path(path=w545) -> (stripped path=w543:path)  [unwired: 1 out]
        }
        frame "Development System", Default {
          n297 = Strip Path(path=w547) -> (stripped path=w546:path)  [unwired: 1 out]
        }
      }
      n298 = Path To String(path=w523) -> (string=w531:string)
      n299 = Concatenate Strings(w531, "\\Reports") -> (w529:string)
      n300 = String To Path(string=w529) -> (path=w527:path)
      n301 = local read "Array"() -> (w533:string[])
      n302 = Index Array(array=w533, index="Reports") -> (element=w532:string)
      n303 = Format Into String(w527) -> (resulting string=w534:string)  [unwired: 3 in, 1 out]
      n304 = case shown="True" "?" {
        tunnel: w527 -> [_ w569]
        tunnel: "Enter ABM Serial Number" -> [_ w567]
        frame False {
        }
        frame True {
          n305 = Equal?(x=w567, y="") -> (x = y?=w570:bool)
          n306 = case shown="False" w570 {
            tunnel: w567 -> [w576 _]
            tunnel: w569 -> [w575 _]
            frame False {
              n307 = Concatenate Strings(w576, "*.TDM" ("string")) -> (w578:string)
              n308 = call <userlib>:"List Directory__ogtk.vi"("pattern"=w578, "directory path"=w575) -> ("file names"=w571:string[])  [unwired: 2 in, 3 out]
              "Array" <- w571
              n309 = property on="Reports" class="LstBox (strict)"("Item Names"=w571) -> ()  [unwired: 2 in, 2 out]
              n310 = Array Size(array=w571) -> (size(s)=w572:i32)
              n311 = Equal?(x=w572, y=0) -> (x = y?=w574:bool)
              n312 = case shown="True" w574 {
                frame False {
                }
                frame True {
                  n313 = One Button Dialog(message="No File Found") -> ()  [unwired: 1 in, 1 out]
                }
              }
            }
            frame True {
              n314 = One Button Dialog(message="Please Enter The ABM Serial") -> ()  [unwired: 1 in, 1 out]
            }
          }
        }
      }
      n315 = Concatenate Strings(w534, "\\" ("string"), w532) -> (w536:string)
      n316 = String To Path(string=w536) -> (path=w539:path)
      n317 = case shown="True" "?" {
        tunnel: w539 -> [_ w551]
        tunnel: w527 -> [_ w550]
        frame False {
        }
        frame True {
          n318 = Equal?(x=w551, y=w550) -> (x = y?=w552:bool)
          n319 = case shown="False" w552 {
            tunnel: w551 -> [w553 _]
            frame False {
              w555 = u16 3 items=["SW_HIDE", "SW_NORMAL", "SW_SHOWMINIMIZED", "SW_SHOWMAXIMIZED", "SW_SHOWNOACTIVATE", "SW_SHOW", "SW_MINIMIZE", "SW_SHOWMINNOACTIVE", "SW_SHOWNA", "SW_RESTORE", "SW_SHOWDEFAULT", "SW_FORCEMINIMIZE"] ("Flag")
              n320 = dll-call lib="user32.dll" fn="GetShellWindow"(error in="error in") -> (error out=w563:errorcluster, w554:u32)  [unwired: 2 in, 1 out]
              n321 = Path To String(path=w553) -> (string=w556:string)
              n322 = dll-call lib="shell32.dll" fn="ShellExecuteA"(error in=w563, "hwnd"=w554, "lpOperation"="open", "lpFile"=w556, "lpParameters"="Parameters", "lpDirectory"="", "nShowCmd"=w555) -> (error out=→"error out 3":errorcluster, w559:i32)  [unwired: 5 in, 4 out]
              "output param" <- w559
              n323 = Less Or Equal?(x=w559, y=32) -> (x <= y?=→"ERROR":bool)
            }
            frame True {
              n324 = One Button Dialog(message="Error, No File Selected, Please Try Again") -> ()  [unwired: 1 in, 1 out]
            }
          }
        }
      }
    }
  }
  n325 = case shown="True" w1 {
    tunnel: w5 -> [_ w614]
    tunnel: w4 -> [_ w583]
    tunnel: w6 -> [_ w613]
    tunnel: w7 -> [_ w581]
    tunnel: w3 -> [_ w591]
    frame False {
    }
    frame True {
      # "range to now if the signal\npassed the test or not"
      n326 = Open Application Reference() -> (3:w587:refnum<vi>)  [unwired: 4 in, 1 out]
      n327 = Format Into String "Format Into String"(w583) -> (resulting string=w623:string)  [unwired: 3 in, 1 out]
      n328 = property class="App"(reference=w587) -> ("App.Kind"=w586:T2)  [unwired: 1 in, 2 out]
      n329 = Current VI's Path() -> (path=w585:path)
      n330 = case shown="\"Run Time System\"" w586 {
        tunnel: w585 -> [w633 w638]
        tunnel: [w634 w637] -> w584
        frame "Run Time System" {
          n331 = Strip Path(path=w633) -> (stripped path=w635:path)  [unwired: 1 out]
          n332 = Strip Path(path=w635) -> (stripped path=w636:path)  [unwired: 1 out]
          n333 = Strip Path(path=w636) -> (stripped path=w634:path)  [unwired: 1 out]
        }
        frame "Development System", Default {
          n334 = Strip Path(path=w638) -> (stripped path=w637:path)  [unwired: 1 out]
        }
      }
      n335 = Concatenate Strings "Concatenate Strings"(w623, " %") -> (w630:string)
      n336 = Path To String(path=w584) -> (string=w599:string)
      n337 = Concatenate Strings(w599, "\\Reports") -> (w592:string)
      n338 = String To Path(string=w592) -> (path=w597:path)
      n339 = local read "Port to test"() -> (w612:u16)
      n340 = call <userlib>:"Create Dir if Non-Existant__ogtk.vi"("Directory Path"=w597) -> ("dup Directory Path"=w596:path)  [unwired: 8 in, 2 out]
      n341 = Increment(x=w612) -> (x+1=w589:u16)
      n342 = Format Into String "Format Into String"(w596) -> (resulting string=w594:string)  [unwired: 3 in, 1 out]
      n343 = Get Date/Time String(date format (0)=enum16{"short", "long", "abbreviated"}."abbreviated") -> (date string=w600:string)  [unwired: 2 in, 1 out]
      n344 = case shown="1, Default" w589 {
        selector: w589 -> [w639 w640 w641 w642 w643 _]
        tunnel: [w639 w640 w641 w642 w643 18] -> w588
        frame 1, Default {
        }
        frame 2 {
        }
        frame 3 {
        }
        frame 4 {
        }
        frame 5 {
        }
        frame 6 {
        }
      }
      n345 = local read "ABM-S/N"() -> (w601:string)
      n346 = Format Into String "Format Into String"(w588) -> (resulting string=w626:string)  [unwired: 3 in, 1 out]
      n347 = Format Into String "Format Into String"(w614) -> (resulting string=w621:string)  [unwired: 3 in, 1 out]
      n348 = Concatenate Strings(w594, "\\" ("string"), w601, " - ", w600, ".tdm") -> (w595:string)
      n349 = String To Path(string=w595) -> (path=w582:path)
      n350 = Concatenate Strings "Concatenate Strings"("Save Data From ", w591) -> (w632:string)
      n351 = String To IP() -> (0:w620:u32)  [unwired: 1 in]
      n352 = IP To String(2:w620) -> (0:w619:string)  [unwired: 1 in]
      n353 = Concatenate Strings "Concatenate Strings"("AMB ", w626, " - " ("string"), w591) -> (w629:string)
      n354 = Concatenate Strings "Concatenate Strings"(w621, " ms") -> (w631:string)
      n355 = local read "Assembled by"() -> (w611:string)
      n356 = xnode "Open Data Storage\n[TDM]"("file path"=w582, "function (open:0)"=T3."open or create") -> ("storage refnum (file)"=w617:refnum<k20>, "error out"=w625:errorcluster)  [unwired: 3 in, 1 out]
      n357 = Get Date/Time In Seconds() -> (seconds since 1Jan1904=w616:timestamp)
      n358 = xnode "Set Properties\n[File]"("Name"=w619, "Description"=w632, "Author"=w611, "Time stamp"=w616, "Date"=w600, "ABM_SerialNumber"=w601, "storage refnum (file)"=w617, "error in"=w625) -> ("storage refnum (file) out"=w627:refnum<k20>, "error out"=w628:errorcluster)
      n359 = xnode "Write Data\n[Channel group]"("Name"=w629, "Description"=w632, "Status"=w613, "Error_Range"=w630, "Periode"=w631, "storage refnum (file)"=w627, "error in"=w628) -> ("error out"=w610:errorcluster, "storage refnum (channel group)"=w609:refnum<k20>)  [unwired: 1 out]
      n360 = xnode "Write Data\n[Channel]"("Signal"=w581, "storage refnum (channel group)"=w609, "error in"=w610) -> ("storage refnum (channel group) out"=w607:refnum<k20>, "error out"=w606:errorcluster)  [unwired: 2 in, 1 out]
      n361 = xnode "Close Data Storage\n"("storage refnum (channel group)"=w607, "error in (no error)"=w606) -> ("error out"=w608:errorcluster)  [unwired: 1 out]
      n362 = call <vilib>:"Simple Error Handler.vi"("error in (no error)"=w608) -> ()  [unwired: 1 in, 8 out]
    }
  }
